vi "Memory Manager Post-Build.vi"   [LabVIEW 2020]
uses:
  Build Automation.lvlib
types:
  T1 = cluster{"Status Message":refnum<data-value>, "Progress":refnum<data-value>, "Stop":refnum<data-value>}
  T2 = enum16{"Share clones between instances", "Preallocate clone for each instance"}
  T3 = enum32{"invalid VI type", "Standard VI", "Control VI", "Global VI", "Polymorphic VI", "Configuration VI", "SubSystem", "Facade VI", "Method VI", "Statechart Diagram VI"}
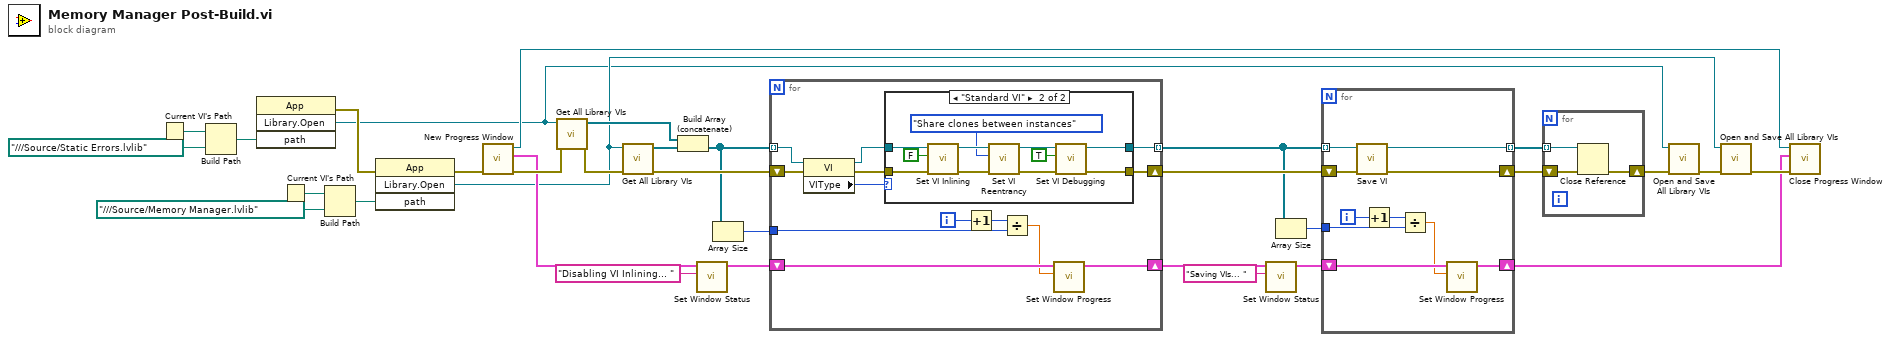
[diagram p0: block diagram]
diagram:
  n1 = Current VI's Path() -> (path=w17:path)
  n2 = Build Path(base path=w17, name or relative path=path "../../../Source/Static Errors.lvlib" ("stripped path")) -> (appended path=w16:path)
  n3 = invoke class="App" method="Library.Open"("path"=w16) -> (error out=w15:errorcluster, "Open Library"=w1:refnum<vi>)  [unwired: 3 in, 2 out]
  n4 = Current VI's Path() -> (path=w19:path)
  n5 = Build Path(base path=w19, name or relative path=path "../../../Source/Memory Manager.lvlib" ("stripped path")) -> (appended path=w33:path)
  n6 = invoke class="App" method="Library.Open"(error in=w15, "path"=w33) -> (error out=w31:errorcluster, "Open Library"=w4:refnum<vi>)  [unwired: 2 in, 2 out]
  n7 = call "New Progress Window.vi"("error in (no error)"=w31) -> ("error out"=w14:errorcluster, "DVRs"=w9:T1, "VI refnum"=w27:refnum<vi>)  [unwired: 8 in]
  n8 = call "Get All Library VIs.vi"("error in (no error)"=w14, "library ref"=w1) -> ("error out"=w13:errorcluster, "vi refs"=w12:refnum<vi>[])  [unwired: 8 in]
  n9 = call "Get All Library VIs.vi"("error in (no error)"=w13, "library ref"=w4) -> ("error out"=w32:errorcluster, "vi refs"=w11:refnum<vi>[])  [unwired: 8 in]
  n10 = Build Array (concatenate)(w12, w11) -> (w10:refnum<vi>[])
  n11 = call "Set Window Status.vi"("Status Message"="Disabling VI Inlining... " ("data value"), "DVRs in"=w9) -> ("DVRs out"=w28:T1)  [unwired: 8 in, 1 out]
  n12 = Array Size(array=w10) -> (size(s)=w29:i32)
  n13 = for {
    tunnel: w10 -> [w38] mode=indexing
    shift-right: [w39] -> w26
    shift-left: w32 -> [w37]
    tunnel: w29 -> [w44]
    shift-right: [w41] -> w25
    shift-left: w28 -> [w43]
    tunnel: [w40] -> w22 mode=indexing
    i -> [w46]
    n14 = property class="VI"(reference=w38, error in=w37) -> (reference out=w36:refnum<vi>, error out=w35:errorcluster, "VIType"=w34:T3)
    n15 = case shown="\"Standard VI\"" w34 {
      tunnel: [w48 w52] -> w40
      tunnel: [w47 w51] -> w39
      tunnel: w36 -> [w48 w50]
      tunnel: w35 -> [w47 w49]
      frame Default {
      }
      frame "Standard VI" {
        n16 = call "Set VI Inlining.vi"("error in (no error)"=w49, "Inline VI"=FALSE, "vi ref in"=w50) -> ("error out"=w56:errorcluster, "vi ref out"=w57:refnum<vi>)  [unwired: 7 in]
        n17 = call "Set VI Reentrancy.vi"("error in (no error)"=w56, "Reentrancy Type"=T2."Share clones between instances", "vi ref in"=w57) -> ("error out"=w53:errorcluster, "vi ref out"=w54:refnum<vi>)  [unwired: 7 in]
        n18 = call "Set VI Debugging.vi"("error in (no error)"=w53, "Allow Debugging"=TRUE, "vi ref in"=w54) -> ("error out"=w51:errorcluster, "vi ref out"=w52:refnum<vi>)  [unwired: 7 in]
      }
    }
    n19 = Increment(x=w46) -> (x+1=w45:i32)
    n20 = Divide(x=w45, y=w44) -> (x/y=w42:dbl)
    n21 = call "Set Window Progress.vi"("Progress"=w42, "DVRs in"=w43) -> ("DVRs out"=w41:T1)  [unwired: 8 in, 1 out]
  }
  n22 = call "Set Window Status.vi"("Status Message"="Saving VIs... ", "DVRs in"=w25) -> ("DVRs out"=w23:T1)  [unwired: 8 in, 1 out]
  n23 = Array Size(array=w22) -> (size(s)=w21:i32)
  n24 = for {
    shift-right: [w67] -> w8
    shift-left: w26 -> [w69]
    tunnel: w22 -> [w68] mode=indexing
    shift-right: [w61] -> w5
    shift-left: w23 -> [w63]
    tunnel: w21 -> [w65]
    tunnel: [w60] -> w7 mode=indexing
    i -> [w64]
    n25 = call "Save VI.vi"("error in (no error)"=w69, "vi ref in"=w68) -> ("error out"=w67:errorcluster, "vi ref out"=w60:refnum<vi>)  [unwired: 8 in]
    n26 = Increment(x=w64) -> (x+1=w66:i32)
    n27 = Divide(x=w66, y=w65) -> (x/y=w62:dbl)
    n28 = call "Set Window Progress.vi"("Progress"=w62, "DVRs in"=w63) -> ("DVRs out"=w61:T1)  [unwired: 8 in, 1 out]
  }
  n29 = for {
    shift-right: [w70] -> w2
    shift-left: w8 -> [w72]
    tunnel: w7 -> [w71] mode=indexing
    n30 = Close Reference(reference=w71, error in (no error)=w72) -> (error out=w70:errorcluster)
  }
  n31 = call "Open and Save All Library VIs.vi"("error in (no error)"=w2, "library ref"=w1) -> ("error out"=w3:errorcluster)  [unwired: 9 in]
  n32 = call "Open and Save All Library VIs.vi"("error in (no error)"=w3, "library ref"=w4) -> ("error out"=w6:errorcluster)  [unwired: 9 in]
  n33 = call "Close Progress Window.vi"("error in (no error)"=w6, "DVRs in"=w5, "VI refnum"=w27) -> ()  [unwired: 8 in, 1 out]
